vi "Merge Libraries.vi"(8 "error in (no error)":errorcluster, 10 "MusicLibrary To Merge":refnum<class "MusicLibrary.lvclass">, 11 "MusicLibrary in":refnum<class "MusicLibrary.lvclass">) -> (0 "error out":errorcluster, 3 "MusicLibrary out":refnum<class "MusicLibrary.lvclass">)   [LabVIEW 2015, in "MusicLibrary.lvclass"]
uses:
  MusicLibrary.lvclass
  MusicElementLibrary.lvclass/MusicElementLibrary.ctl
  MusicElement.lvclass
  MusicElementLibrary.lvclass
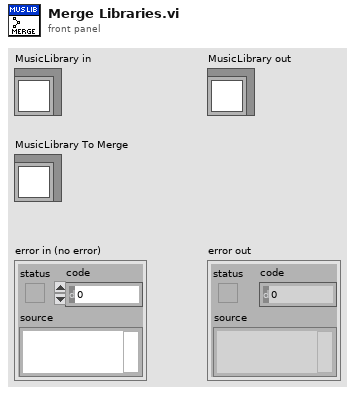
[diagram p1: front panel]
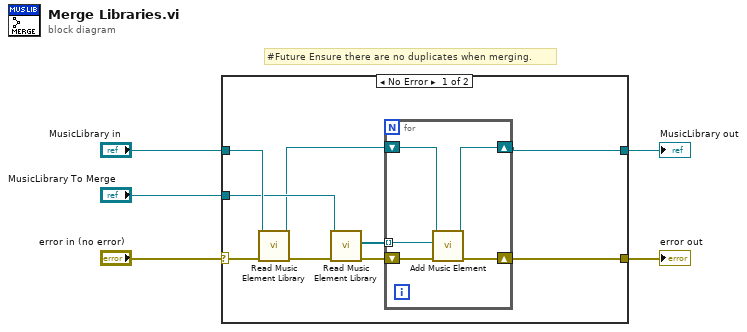
[diagram p0: block diagram]
diagram:
  # "#Future Ensure there are no duplicates when merging."
  n1 = case shown="No Error" "error in (no error)" {
    selector: "error in (no error)" -> [w14 w21]
    tunnel: [w6 w21] -> w4
    tunnel: [w7 w20] -> w2
    tunnel: "MusicLibrary in" -> [w13 w20]
    tunnel: "MusicLibrary To Merge" -> [w11 _]
    frame No Error {
      n2 = call "Read Music Element Library.vi"("error in (no error)"=w14, "MusicElementLibrary in"=w13) -> ("error out"=w12:errorcluster, "MusicElementLibrary out"=w9:refnum<class "MusicLibrary.lvclass">)  [unwired: 7 in, 1 out]
      n3 = call "Read Music Element Library.vi"("error in (no error)"=w12, "MusicElementLibrary in"=w11) -> ("error out"=w10:errorcluster, "Music Element Library"=w8:refnum<class "MusicElement.lvclass">[])  [unwired: 7 in, 1 out]
      n4 = for {
        shift-right: [w15] -> w6
        shift-left: w10 -> [w18]
        shift-right: [w17] -> w7
        shift-left: w9 -> [w19]
        tunnel: w8 -> [w16] mode=indexing
        n5 = call "Add Music Element.vi"("error in (no error)"=w18, "MusicElement"=w16, "MusicElementLibrary in"=w19) -> ("error out"=w15:errorcluster, "MusicElementLibrary out"=w17:refnum<class "MusicLibrary.lvclass">)  [unwired: 7 in]
      }
    }
    frame Error {
    }
  }
  "error out" <- w4
  "MusicLibrary out" <- w2
